vi "MODBUS  SLAVE.vi"() -> (3 "values to write":u16[](array[numeric]) caption="待写入值")   [LabVIEW 2016]
uses:
  <vilib>/NI/Modbus Library/Data Model/Device Data Model.lvclass
  <vilib>/NI/Modbus Library/API/Wrapper/Create TCP Slave.vi
  <vilib>/NI/Modbus Library/API/slave/Modbus Slave.lvclass
  <vilib>/ptbypt/NI_PtbyPt.lvlib
  <vilib>/NI/Modbus Library/API/Wrapper/API Main.lvlib
panel:
  out "运行周期":u16[](array[numeric])
  in  "write operation starting address":u16=100 caption="写操作起始地址"
  out "单仪器启动命令":u16[](array[numeric])
  out "系统启动命令":u16[](array[numeric])
  in  "停止":bool
  out "register values":u16[](array[numeric]) caption="寄存器值"
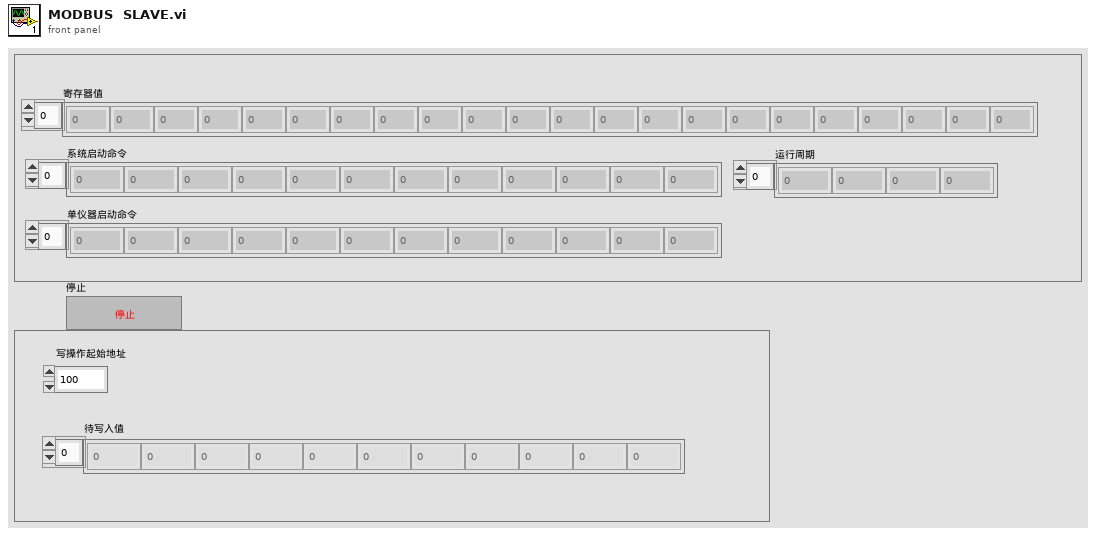
[diagram p1: front panel]
types:
  T1 = cluster{"测量量程":dbl, "测量精度":dbl, "测量间隔":dbl, "消解温度":dbl, "消解时长":dbl, "空白校准时间":timestamp, "曲线截距":dbl, "曲线斜率":dbl, "测量检出限":dbl, "测量信号值":dbl, "线性相关系数":dbl, "二次多项式系数":dbl, "标样校准时间":timestamp, "单位":u16}
  T2 = typedef "LVDateTimeRec.ctl" = cluster{"秒数的小数部分":dbl, "秒":i32, "分":i32, "时":i32, "日":i32, "月":i32, "年":i32, "天数（周）":i32, "天数（年）":i32, "DST":i32}
  T3 = cluster{"时间标识":timestamp, "设备":string, "日志信息":string, "流程参数":string}
  T4 = cluster{"测量模式":enum16{"水样测量", "标样核查", "零点核查", "跨度核查", "空白测试", "加标回收", "平行样", "校零", "校标"}}
  T5 = cluster{"站号":u16, "量程切换":enum32{"H", "L", "AUTO"}, "控制命令":enum16{"启动测量", "标样核查", "零点核查", "跨度核查", "空白测试", "平行样测试", "加标回收", "空白校准", "标样校准", "初始化（清洗）", "停止测试", "仪器重启", "校时", "模式设置", "测量间隔设置"}, "模式设置":enum16{"待机", "连续模式", "周期模式", "定点模式", "受控模式", "手动模式"}, "测量间隔":u16}
  T6 = cluster{"是否启用仪器":bool, "CODMn":cluster{"启动测量模式":cluster{"测量模式":enum16{"水样测量", "标样核查", "加标回收", "平行样", "校零", "校标"}}, "确定按钮":bool}, "启动模块":cluster{"氨氮":bool, "总磷":bool, "总氮":bool, "COD":bool}, "常规启动":bool, "直接启动":bool}
  T7 = cluster{"系统时间":timestamp, "工作状态":enum16{"空闲", "水样测试", "标样核查", "零点核查", "跨度核查", "空白测试", "平行样测试", "加标回收", "空白校准", "标样校准", "初始化（清洗）"}, "测量模式":enum16{"待机", "连续模式", "周期模式", "定点模式", "受控模式", "手动模式"}, "告警代码":u16, "故障代码":u16, "日志代码":u16, "软件版本":u16, "F0":sgl, "F1":sgl, "F2":sgl, "F3":sgl, "T":sgl, "H":sgl, "id":u16, "flowid":u16, "量程":u16, "总磷控温温度1":sgl, "营养盐控温温度2":sgl, "ADC":sgl}
  T8 = enum16{"空闲", "水样测试", "标样核查", "零点核查", "跨度核查", "空白测试", "平行样测试", "质控样", "空白校准", "标样校准", "加标回收"}
  T9 = enum16{"空闲", "水样测试", "标样核查", "零点核查", "跨度核查", "空白测试", "平行样测试", "加标回收", "空白校准", "标样校准", "初始化（清洗）"}
  T10 = cluster{"水样测试量程模式":enum16{"H", "L", "AUTO"}, "空白核查量程模式":enum16{"H", "L", "AUTO"}, "跨度核查量程模式":enum16{"H", "L", "AUTO"}}
  T11 = enum32{"Bad", "Idle", "Run top level", "Running"}
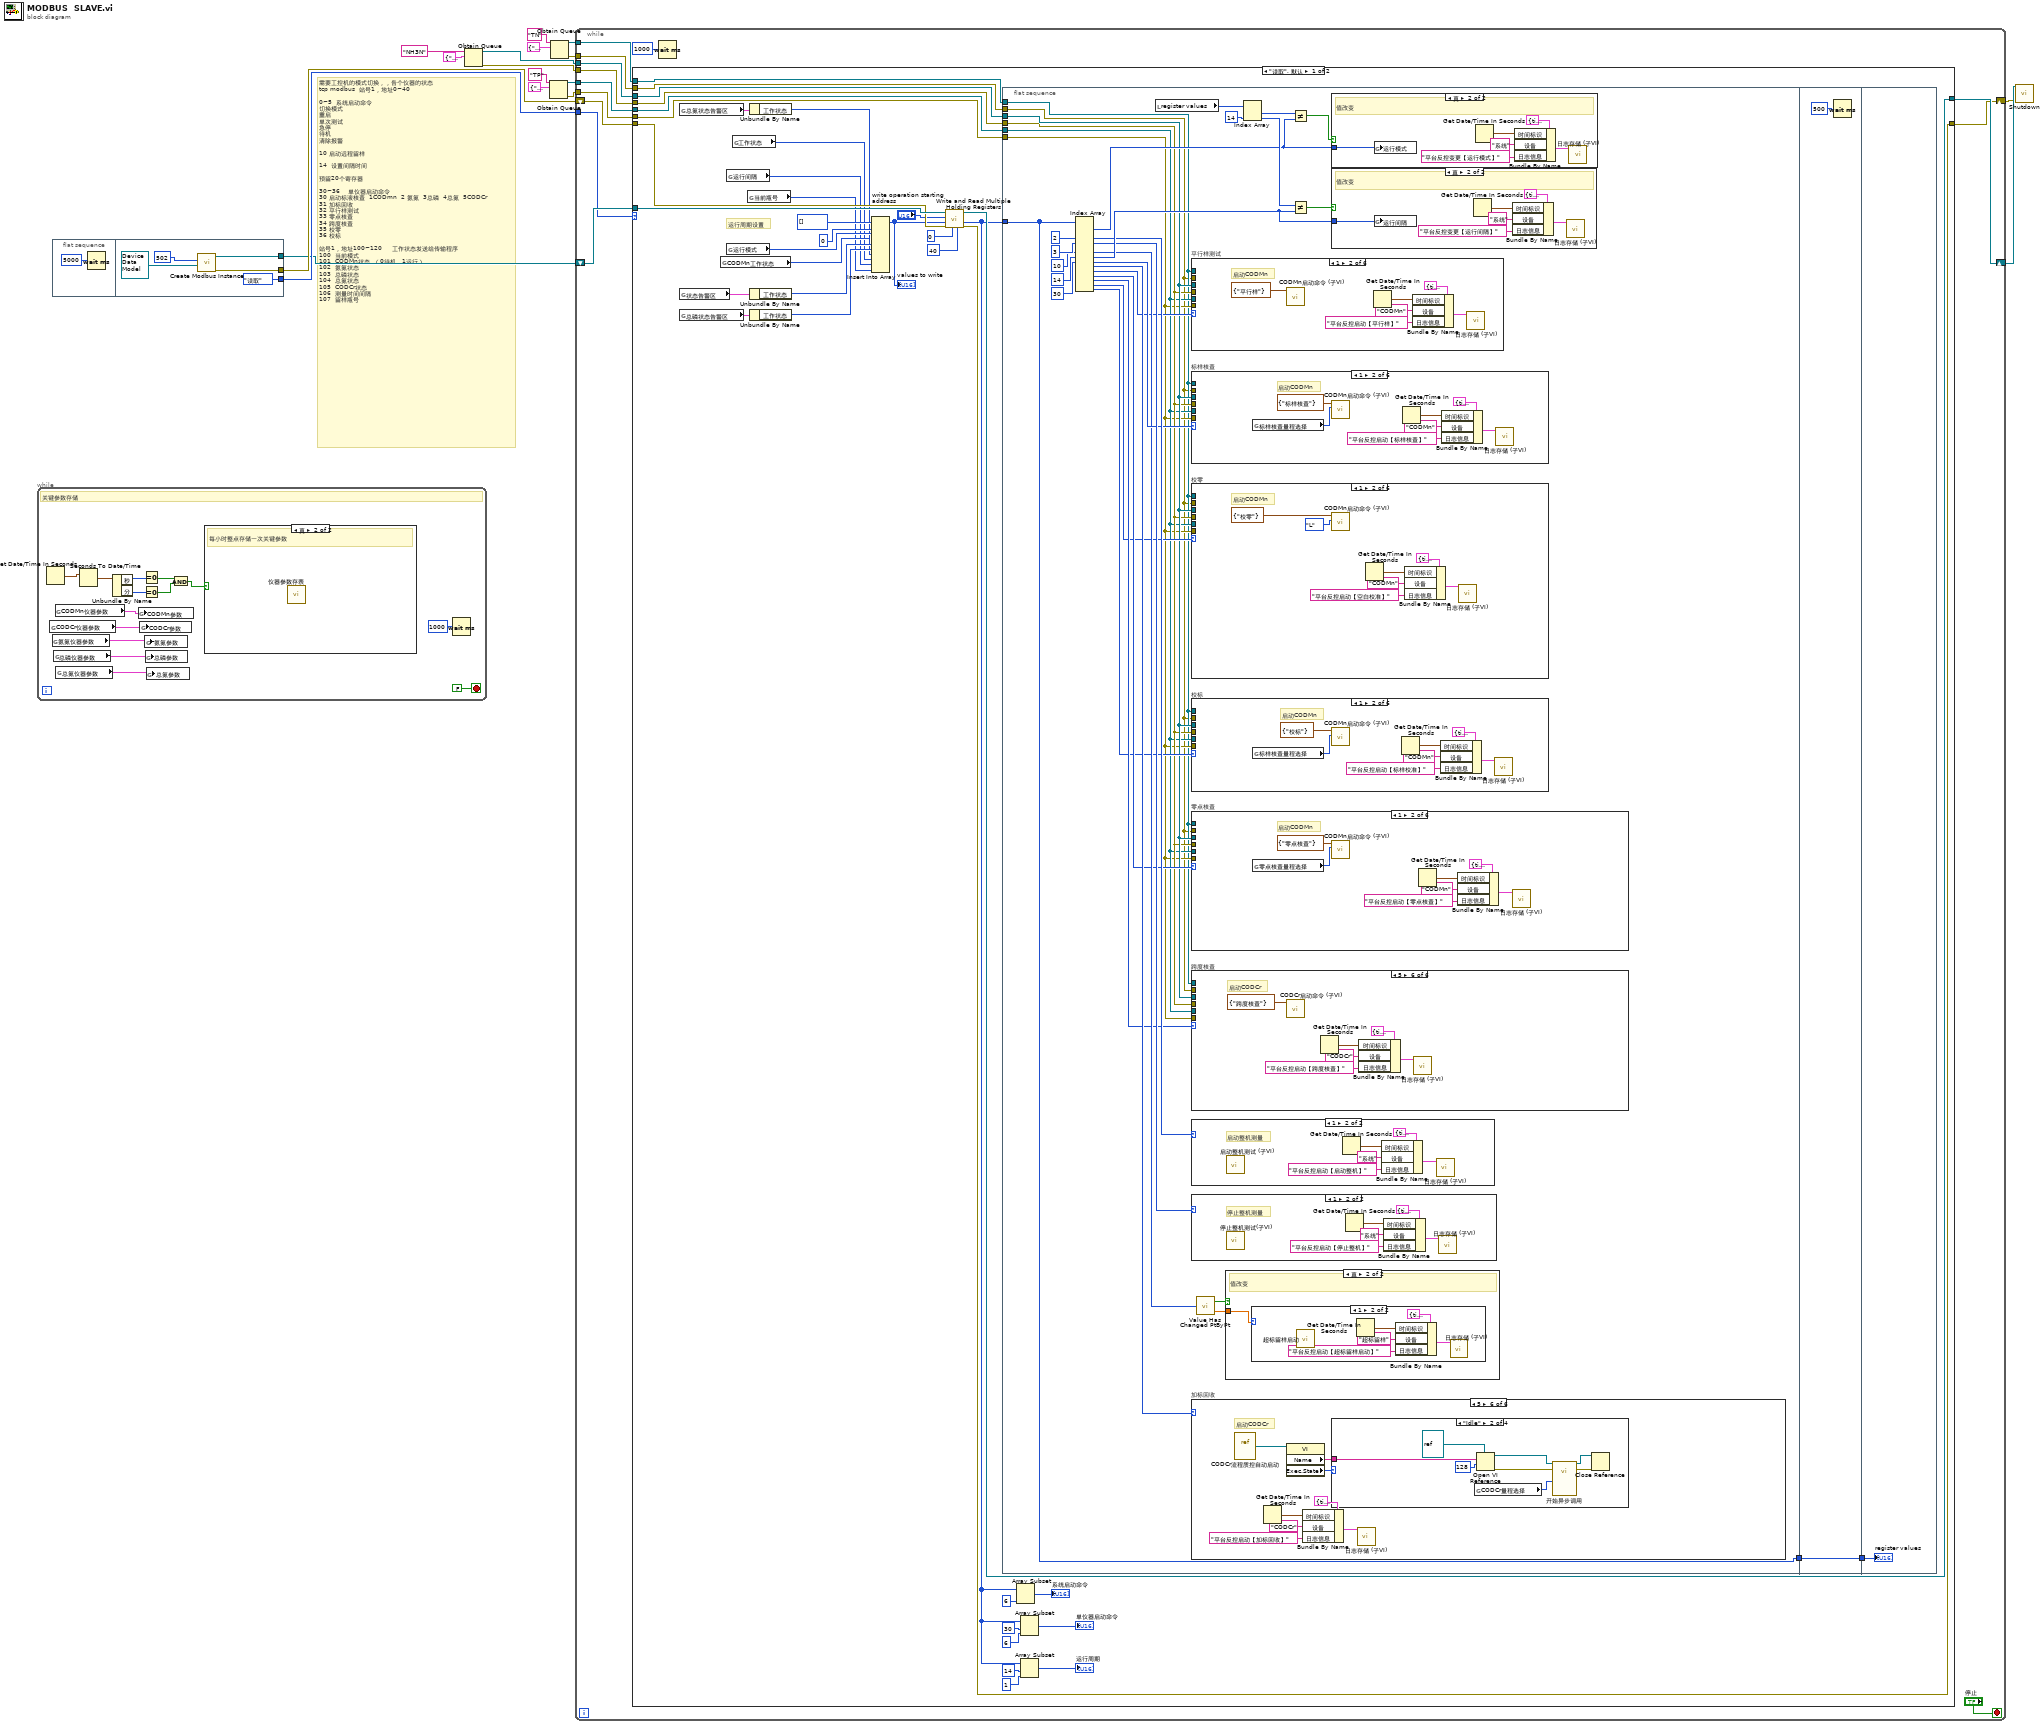
[diagram p0: block diagram]
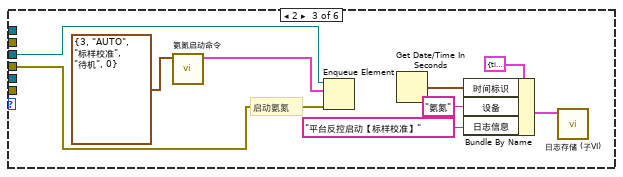
[diagram p4: hidden frame]
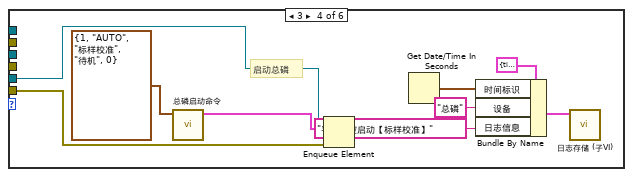
[diagram p5: hidden frame]
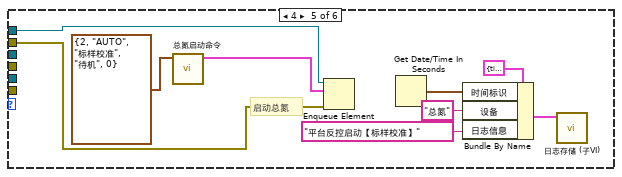
[diagram p6: hidden frame]
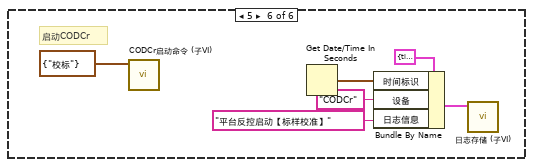
[diagram p7: hidden frame]
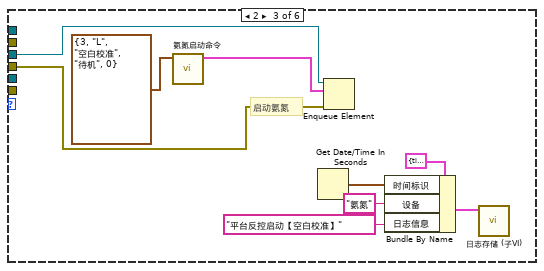
[diagram p9: hidden frame]
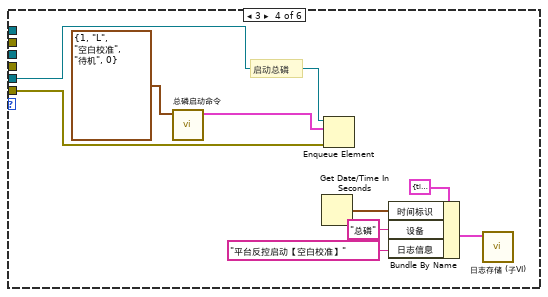
[diagram p10: hidden frame]
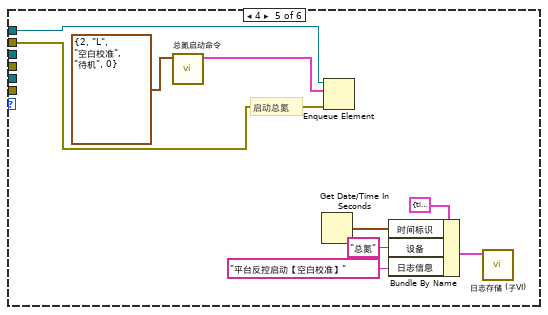
[diagram p11: hidden frame]
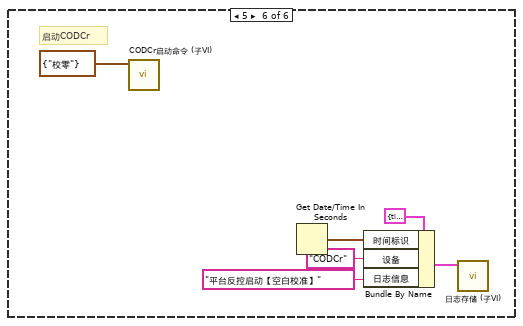
[diagram p12: hidden frame]
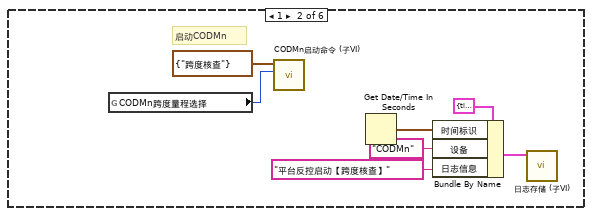
[diagram p14: hidden frame]
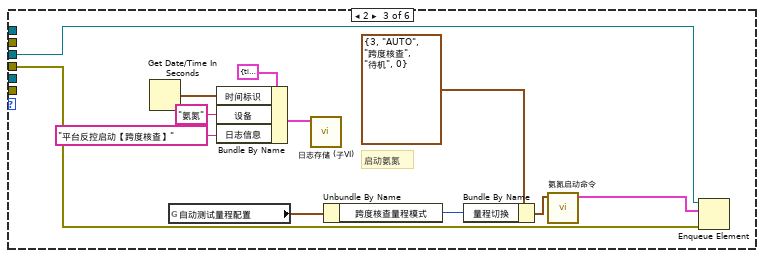
[diagram p15: hidden frame]
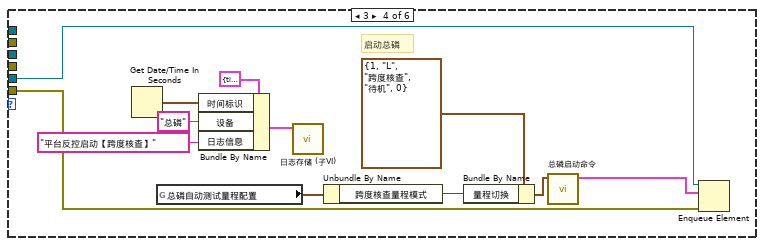
[diagram p16: hidden frame]
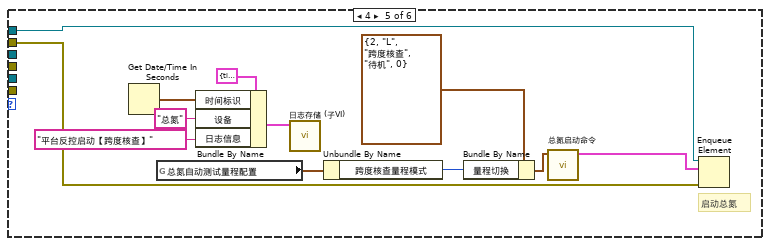
[diagram p17: hidden frame]
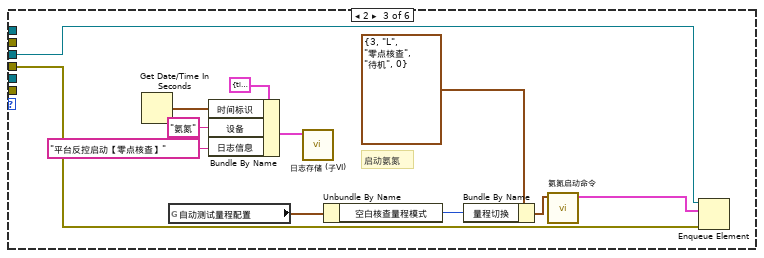
[diagram p19: hidden frame]
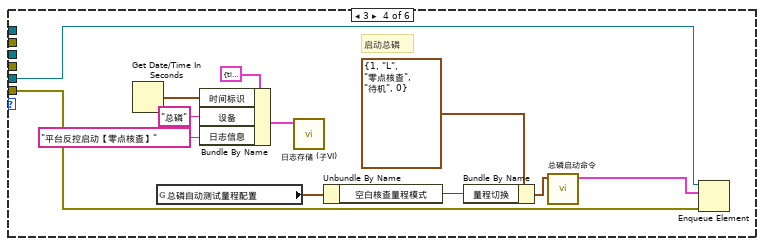
[diagram p20: hidden frame]
diagram:
  # "需要工控机的模式切换，，各个仪器的状态\ntcp modbus  站号1，地址0~40\n\n0~5  系统启动命令\n切换模式\n重启\n单次测试\n急停\n待机\n清除报警\n\n10 启动远程留样\n\n14  设置间隔时间\n\n预留20个寄存器\n\n30~36    单仪器启动命令\n30 启动标液核查  1CODmn  2 氨氮  3总磷  4总氮  5CODCr\n31 加标回收\n32 平行样测试\n33 零点核查\n34 跨度核查\n35 校零\n36 校标\n\n站号1，地址100~120     工作状态发送给传输程序\n100  当前模式\n101  CODMn状态  （0待机，1运行）\n102  氨氮状态\n103  总磷状态\n104  总氮状态\n105  CODCr状态\n106  测量时间间隔\n107  留样瓶号"
  n1 = while {
    stop <- FALSE stop-if-true
    # "关键参数存储"
    n2 = Get Date/Time In Seconds() -> (seconds since 1Jan1904=w29:timestamp)
    n3 = global read "CODcr全局变量.vi" "CODCr仪器参数"() -> (w21:T1)
    n4 = global read "氨氮断电保存全局变量.vi" "氨氮仪器参数"() -> (w20:T1)
    n5 = global read "总磷断电保存全局变量.vi" "总磷仪器参数"() -> (w19:T1)
    n6 = global read "CODMn断电保存全局变量.vi" "CODMn仪器参数"() -> (w22:T1)
    n7 = global read "总氮断电保存全局变量.vi" "总氮仪器参数"() -> (w18:T1)
    n8 = Seconds To Date/Time(time stamp (now)=w29) -> (date time rec=w28:T2)  [unwired: 1 in]
    n9 = Unbundle By Name(w28) -> ("秒"=w27:i32, "分"=w26:i32)
    n10 = global write "在线监测仪器仪表参数.vi" "CODMn参数"(w22) -> ()
    n11 = global write "在线监测仪器仪表参数.vi" "CODCr参数"(w21) -> ()
    n12 = Equal To 0?(x=w27) -> (x = 0?=w25:bool)
    n13 = Equal To 0?(x=w26) -> (x = 0?=w24:bool)
    n14 = global write "在线监测仪器仪表参数.vi" "氨氮参数"(w20) -> ()
    n15 = global write "在线监测仪器仪表参数.vi" "总磷参数"(w19) -> ()
    n16 = global write "在线监测仪器仪表参数.vi" "总氮参数"(w18) -> ()
    n17 = And(x=w25, y=w24) -> (x .and. y?=w23:bool)
    n18 = case shown="真" w23 {
      frame False {
      }
      frame True {
        # "每小时整点存储一次关键参数"
        n19 = call "仪器参数存表.vi"() -> ()  [unwired: 12 in]
      }
    }
    n20 = Wait (ms)(milliseconds to wait=u32 1000 ("等待时间（毫秒）")) -> ()  [unwired: 1 out]
  }
  n21 = flat-sequence {
    tunnel: [enum16{"读取", "写入"}."读取"] -> w17
    tunnel: [w35] -> w16
    tunnel: [w34] -> w15
    frame #0 {
      n22 = Wait (ms)(milliseconds to wait=u32 5000 ("等待时间（毫秒）")) -> ()  [unwired: 1 out]
    }
    frame #1 {
      n23 = call-poly <vilib>:"Create Modbus Instance.vi"("device data model"=refnum<class "Device Data Model.lvclass"> refnum, "port (502)"=u16 502) -> ("error out"=w35:errorcluster, "TCP slave instance"=w34:refnum<class "Modbus Slave.lvclass">)  [unwired: 8 in]
    }
  }
  n24 = Obtain Queue(name (unnamed)="NH3N" ("名称（未命名）"), element data type=cluster{"命令":string, "data":variant} {"命令"="", "data"=variant}) -> (queue out=w6:refnum<queue>, error out=w5:errorcluster)  [unwired: 3 in, 1 out]
  n25 = Obtain Queue(name (unnamed)="TP" ("名称（未命名）"), element data type=cluster{"命令":string, "data":variant} {"命令"="", "data"=variant}) -> (queue out=w4:refnum<queue>, error out=w3:errorcluster)  [unwired: 3 in, 1 out]
  n26 = Obtain Queue(name (unnamed)="TN" ("名称（未命名）"), element data type=cluster{"命令":string, "data":variant} {"命令"="", "data"=variant}) -> (queue out=w2:refnum<queue>, error out=w1:errorcluster)  [unwired: 3 in, 1 out]
  n27 = while {
    shift-right: [w48] -> w14
    shift-left: w15 -> [w50]
    shift-right: [w44] -> w13
    shift-left: w16 -> [w49]
    tunnel: w17 -> [w45]
    tunnel: w6 -> [w43]
    tunnel: w5 -> [w42]
    tunnel: w4 -> [w41]
    tunnel: w3 -> [w40]
    tunnel: w2 -> [w39]
    tunnel: w1 -> [w38]
    stop <- "停止" stop-if-true
    n28 = case shown="\"读取\", 默认" w45 {
      tunnel: w50 -> [w84 w498]
      tunnel: w49 -> [w83 w497]
      tunnel: [w79 w498] -> w48
      tunnel: [w80 w497] -> w44
      tunnel: w43 -> [w56 _]
      tunnel: w42 -> [w55 _]
      tunnel: w41 -> [w54 _]
      tunnel: w40 -> [w53 _]
      tunnel: w39 -> [w52 _]
      tunnel: w38 -> [w51 _]
      frame "读取", Default {
        # "运行周期设置"
        n29 = global read "VAR总磷全局变量.vi" "总氮状态告警区"() -> (w62:T7)
        n30 = global read "VAR氨氮全局变量.vi" "状态告警区"() -> (w66:T7)
        n31 = global read "VAR总磷全局变量.vi" "总磷状态告警区"() -> (w64:T7)
        n32 = global read "COD测量模式全局.vi" "CODMn工作状态"() -> (w60:T8)
        n33 = global read "系统设置全局变量.vi" "运行间隔"() -> (w58:i16)
        n34 = global read "系统设置全局变量.vi" "运行模式"() -> (w76:enum16{"维护模式", "常规模式", "应急模式", "质控模式"})
        n35 = global read "CODcr全局变量.vi" "工作状态"() -> (w59:T9)
        n36 = global read "超标留样全局.vi" "当前瓶号"() -> (w57:u16)
        n37 = Unbundle By Name(w62) -> ("工作状态"=w61:T9)
        n38 = Unbundle By Name(w66) -> ("工作状态"=w65:T9)
        n39 = Unbundle By Name(w64) -> ("工作状态"=w63:T9)
        n40 = Insert Into Array(array=u16[] [] ("values to write"), index=0 ("索引"), new element #1=w76, new element #2=w60, new element #3=w65, new element #4=w63, new element #5=w61, new element #6=w59, new element #7=w58, new element #8=w57) -> (w74:u16[])
        "values to write" <- w74
        n41 = call-dynamic "Write and Read Multiple Holding Registers.vi"("read count"=u16 40 ("number of holding registers"), "read starting address"=u16 0 ("starting address"), "error in"=w83, "write values"=w74, "write starting address"="write operation starting address", "Modbus instance in"=w84) -> ("error out"=w80:errorcluster, "read values"=w69:u16[], "Modbus instance out"=w79:refnum<class "Modbus Slave.lvclass">)  [unwired: 3 in]
        n42 = flat-sequence {
          tunnel: w69 -> [w120]
          tunnel: [w120] -> w68
          tunnel: w56 -> [w94]
          tunnel: w55 -> [w93]
          tunnel: w54 -> [w92]
          tunnel: w53 -> [w91]
          tunnel: w52 -> [w90]
          tunnel: w51 -> [w89]
          tunnel: w68 -> [w494]
          tunnel: [w494] -> w67
          tunnel: w67 -> [w496]
          frame #0 {
            n43 = Index Array(array=w120, index #3=2 ("索引"), index #4=3 ("索引"), index #6=10 ("索引"), index #7=14 ("索引"), index #8=30 ("索引")) -> (element #1=w107:u16, element #3=w108:u16, element #4=w109:u16, element #6=w102:u16, element #7=w110:u16, element #8=w105:u16, element #9=w104:u16, element #10=w99:u16, element #11=w98:u16, element #12=w97:u16, element #13=w96:u16, element #14=w95:u16)  [unwired: 9 in, 2 out]
            n44 = local read "register values"() -> (w119:u16[])
            n45 = case "平行样测试" shown="1" w99 {
              tunnel: w94 -> [_ _ w311 _ _ _]
              tunnel: w93 -> [_ _ w310 _ _ _]
              tunnel: w92 -> [_ _ _ w320 _ _]
              tunnel: w91 -> [_ _ _ w319 _ _]
              tunnel: w90 -> [_ _ _ _ w329 _]
              tunnel: w89 -> [_ _ _ _ w328 _]
              frame 0, Default {
              }
              frame 1 {
                # "启动CODMn"
                n46 = call "CODMn启动命令 (子VI).vi"("启动测量模式"=T4 {"测量模式"=enum."平行样"}) -> ()  [unwired: 11 in]
                n47 = Get Date/Time In Seconds() -> (seconds since 1Jan1904=w301:timestamp)
                n48 = Bundle By Name(cluster=T3 {"时间标识"=timestamp(0 s since 1904-01-01), "设备"="", "日志信息"="", "流程参数"=""} ("data in"), "时间标识"=w301, "设备"="CODMn", "日志信息"="平台反控启动【平行样】") -> (w302:T3)
                n49 = call "日志存储 (子VI).vi"("data in"=w302) -> ()  [unwired: 11 in]
              }
              frame 2 {
                # "启动氨氮"
                n50 = call "氨氮启动命令.vi"("参数"=T5 {"站号"=3, "量程切换"=enum."AUTO", "控制命令"=enum."平行样测试", "模式设置"=enum."待机", "测量间隔"=0}) -> ("启动命令"=w312:cluster{"命令":string, "data":variant})  [unwired: 10 in]
                n51 = Get Date/Time In Seconds() -> (seconds since 1Jan1904=w307:timestamp)
                n52 = Bundle By Name(cluster=T3 {"时间标识"=timestamp(0 s since 1904-01-01), "设备"="", "日志信息"="", "流程参数"=""} ("data in"), "时间标识"=w307, "设备"="氨氮", "日志信息"="平台反控启动【平行样】") -> (w308:T3)
                n53 = Enqueue Element(queue=w311, element=w312, error in (no error)=w310) -> ()  [unwired: 1 in, 3 out]
                n54 = call "日志存储 (子VI).vi"("data in"=w308) -> ()  [unwired: 11 in]
              }
              frame 3 {
                # "启动总磷"
                n55 = call "总磷启动命令.vi"("参数"=T5 {"站号"=1, "量程切换"=enum."AUTO", "控制命令"=enum."平行样测试", "模式设置"=enum."待机", "测量间隔"=0}) -> ("启动命令"=w321:cluster{"命令":string, "data":variant})  [unwired: 10 in]
                n56 = Get Date/Time In Seconds() -> (seconds since 1Jan1904=w316:timestamp)
                n57 = Bundle By Name(cluster=T3 {"时间标识"=timestamp(0 s since 1904-01-01), "设备"="", "日志信息"="", "流程参数"=""} ("data in"), "时间标识"=w316, "设备"="总磷", "日志信息"="平台反控启动【平行样】") -> (w317:T3)
                n58 = Enqueue Element(queue=w320, element=w321, error in (no error)=w319) -> ()  [unwired: 1 in, 3 out]
                n59 = call "日志存储 (子VI).vi"("data in"=w317) -> ()  [unwired: 11 in]
              }
              frame 4 {
                # "启动总氮"
                n60 = call "总氮启动命令.vi"("参数"=T5 {"站号"=2, "量程切换"=enum."AUTO", "控制命令"=enum."平行样测试", "模式设置"=enum."待机", "测量间隔"=0}) -> ("启动命令"=w330:cluster{"命令":string, "data":variant})  [unwired: 10 in]
                n61 = Get Date/Time In Seconds() -> (seconds since 1Jan1904=w325:timestamp)
                n62 = Bundle By Name(cluster=T3 {"时间标识"=timestamp(0 s since 1904-01-01), "设备"="", "日志信息"="", "流程参数"=""} ("data in"), "时间标识"=w325, "设备"="总氮", "日志信息"="平台反控启动【平行样】") -> (w326:T3)
                n63 = Enqueue Element(queue=w329, element=w330, error in (no error)=w328) -> ()  [unwired: 1 in, 3 out]
                n64 = call "日志存储 (子VI).vi"("data in"=w326) -> ()  [unwired: 11 in]
              }
              frame 5 {
                # "启动CODCr"
                n65 = call "CODCr启动命令 (子VI).vi"("启动测量模式"=T4 {"测量模式"=enum."平行样"}) -> ()  [unwired: 11 in]
                n66 = Get Date/Time In Seconds() -> (seconds since 1Jan1904=w334:timestamp)
                n67 = Bundle By Name(cluster=T3 {"时间标识"=timestamp(0 s since 1904-01-01), "设备"="", "日志信息"="", "流程参数"=""} ("data in"), "时间标识"=w334, "设备"="CODCr", "日志信息"="平台反控启动【平行样】") -> (w335:T3)
                n68 = call "日志存储 (子VI).vi"("data in"=w335) -> ()  [unwired: 11 in]
              }
            }
            n69 = case "标样核查" shown="1" w105 {
              tunnel: w94 -> [_ _ w445 _ _ _]
              tunnel: w93 -> [_ _ w444 _ _ _]
              tunnel: w92 -> [_ _ _ w454 _ _]
              tunnel: w91 -> [_ _ _ w453 _ _]
              tunnel: w90 -> [_ _ _ _ w463 _]
              tunnel: w89 -> [_ _ _ _ w462 _]
              frame 0, Default {
              }
              frame 1 {
                # "启动CODMn"
                n70 = global read "CODMn断电保存全局变量.vi" "标样核查量程选择"() -> (w437:enum32{"H", "L", "AUTO"})
                n71 = call "CODMn启动命令 (子VI).vi"("CODMn量程切换"=w437, "启动测量模式"=T4 {"测量模式"=enum."标样核查"}) -> ()  [unwired: 10 in]
                n72 = Get Date/Time In Seconds() -> (seconds since 1Jan1904=w434:timestamp)
                n73 = Bundle By Name(cluster=T3 {"时间标识"=timestamp(0 s since 1904-01-01), "设备"="", "日志信息"="", "流程参数"=""} ("data in"), "时间标识"=w434, "设备"="CODMn", "日志信息"="平台反控启动【标样核查】") -> (w435:T3)
                n74 = call "日志存储 (子VI).vi"("data in"=w435) -> ()  [unwired: 11 in]
              }
              frame 2 {
                # "启动氨氮"
                n75 = call "氨氮启动命令.vi"("参数"=T5 {"站号"=3, "量程切换"=enum."AUTO", "控制命令"=enum."标样核查", "模式设置"=enum."待机", "测量间隔"=0}) -> ("启动命令"=w446:cluster{"命令":string, "data":variant})  [unwired: 10 in]
                n76 = Enqueue Element(queue=w445, element=w446, error in (no error)=w444) -> ()  [unwired: 1 in, 3 out]
                n77 = Get Date/Time In Seconds() -> (seconds since 1Jan1904=w441:timestamp)
                n78 = Bundle By Name(cluster=T3 {"时间标识"=timestamp(0 s since 1904-01-01), "设备"="", "日志信息"="", "流程参数"=""} ("data in"), "时间标识"=w441, "设备"="氨氮", "日志信息"="平台反控启动【标样核查】") -> (w442:T3)
                n79 = call "日志存储 (子VI).vi"("data in"=w442) -> ()  [unwired: 11 in]
              }
              frame 3 {
                # "启动总磷"
                n80 = call "总磷启动命令.vi"("参数"=T5 {"站号"=1, "量程切换"=enum."AUTO", "控制命令"=enum."标样核查", "模式设置"=enum."待机", "测量间隔"=0}) -> ("启动命令"=w455:cluster{"命令":string, "data":variant})  [unwired: 10 in]
                n81 = Enqueue Element(queue=w454, element=w455, error in (no error)=w453) -> ()  [unwired: 1 in, 3 out]
                n82 = Get Date/Time In Seconds() -> (seconds since 1Jan1904=w450:timestamp)
                n83 = Bundle By Name(cluster=T3 {"时间标识"=timestamp(0 s since 1904-01-01), "设备"="", "日志信息"="", "流程参数"=""} ("data in"), "时间标识"=w450, "设备"="总磷", "日志信息"="平台反控启动【标样核查】") -> (w451:T3)
                n84 = call "日志存储 (子VI).vi"("data in"=w451) -> ()  [unwired: 11 in]
              }
              frame 4 {
                # "启动总氮"
                n85 = call "总氮启动命令.vi"("参数"=T5 {"站号"=2, "量程切换"=enum."AUTO", "控制命令"=enum."标样核查", "模式设置"=enum."待机", "测量间隔"=0}) -> ("启动命令"=w464:cluster{"命令":string, "data":variant})  [unwired: 10 in]
                n86 = Enqueue Element(queue=w463, element=w464, error in (no error)=w462) -> ()  [unwired: 1 in, 3 out]
                n87 = Get Date/Time In Seconds() -> (seconds since 1Jan1904=w459:timestamp)
                n88 = Bundle By Name(cluster=T3 {"时间标识"=timestamp(0 s since 1904-01-01), "设备"="", "日志信息"="", "流程参数"=""} ("data in"), "时间标识"=w459, "设备"="总氮", "日志信息"="平台反控启动【标样核查】") -> (w460:T3)
                n89 = call "日志存储 (子VI).vi"("data in"=w460) -> ()  [unwired: 11 in]
              }
              frame 5 {
                # "启动CODCr"
                n90 = call "CODCr启动命令 (子VI).vi"("启动测量模式"=T4 {"测量模式"=enum."标样核查"}) -> ()  [unwired: 11 in]
                n91 = Get Date/Time In Seconds() -> (seconds since 1Jan1904=w468:timestamp)
                n92 = Bundle By Name(cluster=T3 {"时间标识"=timestamp(0 s since 1904-01-01), "设备"="", "日志信息"="", "流程参数"=""} ("data in"), "时间标识"=w468, "设备"="CODCr", "日志信息"="平台反控启动【标样核查】") -> (w469:T3)
                n93 = call "日志存储 (子VI).vi"("data in"=w469) -> ()  [unwired: 11 in]
              }
            }
            n94 = case "校零" shown="1" w96 {
              tunnel: w94 -> [_ _ w174 _ _ _]
              tunnel: w93 -> [_ _ w173 _ _ _]
              tunnel: w92 -> [_ _ _ w183 _ _]
              tunnel: w91 -> [_ _ _ w182 _ _]
              tunnel: w90 -> [_ _ _ _ w192 _]
              tunnel: w89 -> [_ _ _ _ w191 _]
              frame 0, Default {
              }
              frame 1 {
                # "启动CODMn"
                n95 = call "CODMn启动命令 (子VI).vi"("CODMn量程切换"=enum32{"H", "L", "AUTO"}."L", "启动测量模式"=T4 {"测量模式"=enum."校零"}) -> ()  [unwired: 10 in]
                n96 = Get Date/Time In Seconds() -> (seconds since 1Jan1904=w163:timestamp)
                n97 = Bundle By Name(cluster=T3 {"时间标识"=timestamp(0 s since 1904-01-01), "设备"="", "日志信息"="", "流程参数"=""} ("data in"), "时间标识"=w163, "设备"="CODMn", "日志信息"="平台反控启动【空白校准】") -> (w164:T3)
                n98 = call "日志存储 (子VI).vi"("data in"=w164) -> ()  [unwired: 11 in]
              }
              frame 2 {
                # "启动氨氮"
                n99 = call "氨氮启动命令.vi"("参数"=T5 {"站号"=3, "量程切换"=enum."L", "控制命令"=enum."空白校准", "模式设置"=enum."待机", "测量间隔"=0}) -> ("启动命令"=w175:cluster{"命令":string, "data":variant})  [unwired: 10 in]
                n100 = Get Date/Time In Seconds() -> (seconds since 1Jan1904=w170:timestamp)
                n101 = Enqueue Element(queue=w174, element=w175, error in (no error)=w173) -> ()  [unwired: 1 in, 3 out]
                n102 = Bundle By Name(cluster=T3 {"时间标识"=timestamp(0 s since 1904-01-01), "设备"="", "日志信息"="", "流程参数"=""} ("data in"), "时间标识"=w170, "设备"="氨氮", "日志信息"="平台反控启动【空白校准】") -> (w171:T3)
                n103 = call "日志存储 (子VI).vi"("data in"=w171) -> ()  [unwired: 11 in]
              }
              frame 3 {
                # "启动总磷"
                n104 = call "总磷启动命令.vi"("参数"=T5 {"站号"=1, "量程切换"=enum."L", "控制命令"=enum."空白校准", "模式设置"=enum."待机", "测量间隔"=0}) -> ("启动命令"=w184:cluster{"命令":string, "data":variant})  [unwired: 10 in]
                n105 = Get Date/Time In Seconds() -> (seconds since 1Jan1904=w179:timestamp)
                n106 = Enqueue Element(queue=w183, element=w184, error in (no error)=w182) -> ()  [unwired: 1 in, 3 out]
                n107 = Bundle By Name(cluster=T3 {"时间标识"=timestamp(0 s since 1904-01-01), "设备"="", "日志信息"="", "流程参数"=""} ("data in"), "时间标识"=w179, "设备"="总磷", "日志信息"="平台反控启动【空白校准】") -> (w180:T3)
                n108 = call "日志存储 (子VI).vi"("data in"=w180) -> ()  [unwired: 11 in]
              }
              frame 4 {
                # "启动总氮"
                n109 = call "总氮启动命令.vi"("参数"=T5 {"站号"=2, "量程切换"=enum."L", "控制命令"=enum."空白校准", "模式设置"=enum."待机", "测量间隔"=0}) -> ("启动命令"=w193:cluster{"命令":string, "data":variant})  [unwired: 10 in]
                n110 = Get Date/Time In Seconds() -> (seconds since 1Jan1904=w188:timestamp)
                n111 = Enqueue Element(queue=w192, element=w193, error in (no error)=w191) -> ()  [unwired: 1 in, 3 out]
                n112 = Bundle By Name(cluster=T3 {"时间标识"=timestamp(0 s since 1904-01-01), "设备"="", "日志信息"="", "流程参数"=""} ("data in"), "时间标识"=w188, "设备"="总氮", "日志信息"="平台反控启动【空白校准】") -> (w189:T3)
                n113 = call "日志存储 (子VI).vi"("data in"=w189) -> ()  [unwired: 11 in]
              }
              frame 5 {
                # "启动CODCr"
                n114 = call "CODCr启动命令 (子VI).vi"("启动测量模式"=T4 {"测量模式"=enum."校零"}) -> ()  [unwired: 11 in]
                n115 = Get Date/Time In Seconds() -> (seconds since 1Jan1904=w197:timestamp)
                n116 = Bundle By Name(cluster=T3 {"时间标识"=timestamp(0 s since 1904-01-01), "设备"="", "日志信息"="", "流程参数"=""} ("data in"), "时间标识"=w197, "设备"="CODCr", "日志信息"="平台反控启动【空白校准】") -> (w198:T3)
                n117 = call "日志存储 (子VI).vi"("data in"=w198) -> ()  [unwired: 11 in]
              }
            }
            n118 = case "校标" shown="1" w95 {
              tunnel: w94 -> [_ _ w134 _ _ _]
              tunnel: w93 -> [_ _ w133 _ _ _]
              tunnel: w92 -> [_ _ _ w143 _ _]
              tunnel: w91 -> [_ _ _ w142 _ _]
              tunnel: w90 -> [_ _ _ _ w152 _]
              tunnel: w89 -> [_ _ _ _ w151 _]
              frame 0, Default {
              }
              frame 1 {
                # "启动CODMn"
                n119 = global read "CODMn断电保存全局变量.vi" "标样核查量程选择"() -> (w126:enum32{"H", "L", "AUTO"})
                n120 = call "CODMn启动命令 (子VI).vi"("CODMn量程切换"=w126, "启动测量模式"=T4 {"测量模式"=enum."校标"}) -> ()  [unwired: 10 in]
                n121 = Get Date/Time In Seconds() -> (seconds since 1Jan1904=w123:timestamp)
                n122 = Bundle By Name(cluster=T3 {"时间标识"=timestamp(0 s since 1904-01-01), "设备"="", "日志信息"="", "流程参数"=""} ("data in"), "时间标识"=w123, "设备"="CODMn", "日志信息"="平台反控启动【标样校准】") -> (w124:T3)
                n123 = call "日志存储 (子VI).vi"("data in"=w124) -> ()  [unwired: 11 in]
              }
              frame 2 {
                # "启动氨氮"
                n124 = call "氨氮启动命令.vi"("参数"=T5 {"站号"=3, "量程切换"=enum."AUTO", "控制命令"=enum."标样校准", "模式设置"=enum."待机", "测量间隔"=0}) -> ("启动命令"=w135:cluster{"命令":string, "data":variant})  [unwired: 10 in]
                n125 = Enqueue Element(queue=w134, element=w135, error in (no error)=w133) -> ()  [unwired: 1 in, 3 out]
                n126 = Get Date/Time In Seconds() -> (seconds since 1Jan1904=w130:timestamp)
                n127 = Bundle By Name(cluster=T3 {"时间标识"=timestamp(0 s since 1904-01-01), "设备"="", "日志信息"="", "流程参数"=""} ("data in"), "时间标识"=w130, "设备"="氨氮", "日志信息"="平台反控启动【标样校准】") -> (w131:T3)
                n128 = call "日志存储 (子VI).vi"("data in"=w131) -> ()  [unwired: 11 in]
              }
              frame 3 {
                # "启动总磷"
                n129 = call "总磷启动命令.vi"("参数"=T5 {"站号"=1, "量程切换"=enum."AUTO", "控制命令"=enum."标样校准", "模式设置"=enum."待机", "测量间隔"=0}) -> ("启动命令"=w144:cluster{"命令":string, "data":variant})  [unwired: 10 in]
                n130 = Enqueue Element(queue=w143, element=w144, error in (no error)=w142) -> ()  [unwired: 1 in, 3 out]
                n131 = Get Date/Time In Seconds() -> (seconds since 1Jan1904=w139:timestamp)
                n132 = Bundle By Name(cluster=T3 {"时间标识"=timestamp(0 s since 1904-01-01), "设备"="", "日志信息"="", "流程参数"=""} ("data in"), "时间标识"=w139, "设备"="总磷", "日志信息"="平台反控启动【标样校准】") -> (w140:T3)
                n133 = call "日志存储 (子VI).vi"("data in"=w140) -> ()  [unwired: 11 in]
              }
              frame 4 {
                # "启动总氮"
                n134 = call "总氮启动命令.vi"("参数"=T5 {"站号"=2, "量程切换"=enum."AUTO", "控制命令"=enum."标样校准", "模式设置"=enum."待机", "测量间隔"=0}) -> ("启动命令"=w153:cluster{"命令":string, "data":variant})  [unwired: 10 in]
                n135 = Enqueue Element(queue=w152, element=w153, error in (no error)=w151) -> ()  [unwired: 1 in, 3 out]
                n136 = Get Date/Time In Seconds() -> (seconds since 1Jan1904=w148:timestamp)
                n137 = Bundle By Name(cluster=T3 {"时间标识"=timestamp(0 s since 1904-01-01), "设备"="", "日志信息"="", "流程参数"=""} ("data in"), "时间标识"=w148, "设备"="总氮", "日志信息"="平台反控启动【标样校准】") -> (w149:T3)
                n138 = call "日志存储 (子VI).vi"("data in"=w149) -> ()  [unwired: 11 in]
              }
              frame 5 {
                # "启动CODCr"
                n139 = call "CODCr启动命令 (子VI).vi"("启动测量模式"=T4 {"测量模式"=enum."校标"}) -> ()  [unwired: 11 in]
                n140 = Get Date/Time In Seconds() -> (seconds since 1Jan1904=w157:timestamp)
                n141 = Bundle By Name(cluster=T3 {"时间标识"=timestamp(0 s since 1904-01-01), "设备"="", "日志信息"="", "流程参数"=""} ("data in"), "时间标识"=w157, "设备"="CODCr", "日志信息"="平台反控启动【标样校准】") -> (w158:T3)
                n142 = call "日志存储 (子VI).vi"("data in"=w158) -> ()  [unwired: 11 in]
              }
            }
            n143 = case "零点核查" shown="1" w98 {
              tunnel: w94 -> [_ _ w267 _ _ _]
              tunnel: w93 -> [_ _ w266 _ _ _]
              tunnel: w92 -> [_ _ _ w279 _ _]
              tunnel: w91 -> [_ _ _ w278 _ _]
              tunnel: w90 -> [_ _ _ _ w291 _]
              tunnel: w89 -> [_ _ _ _ w290 _]
              frame 0, Default {
              }
              frame 1 {
                # "启动CODMn"
                n144 = global read "CODMn断电保存全局变量.vi" "零点核查量程选择"() -> (w255:enum32{"H", "L", "AUTO"})
                n145 = call "CODMn启动命令 (子VI).vi"("CODMn量程切换"=w255, "启动测量模式"=T4 {"测量模式"=enum."零点核查"}) -> ()  [unwired: 10 in]
                n146 = Get Date/Time In Seconds() -> (seconds since 1Jan1904=w252:timestamp)
                n147 = Bundle By Name(cluster=T3 {"时间标识"=timestamp(0 s since 1904-01-01), "设备"="", "日志信息"="", "流程参数"=""} ("data in"), "时间标识"=w252, "设备"="CODMn", "日志信息"="平台反控启动【零点核查】") -> (w253:T3)
                n148 = call "日志存储 (子VI).vi"("data in"=w253) -> ()  [unwired: 11 in]
              }
              frame 2 {
                # "启动氨氮"
                n149 = Get Date/Time In Seconds() -> (seconds since 1Jan1904=w259:timestamp)
                n150 = global read "氨氮断电保存全局变量.vi" "自动测试量程配置"() -> (w265:T10)
                n151 = Bundle By Name(cluster=T3 {"时间标识"=timestamp(0 s since 1904-01-01), "设备"="", "日志信息"="", "流程参数"=""} ("data in"), "时间标识"=w259, "设备"="氨氮", "日志信息"="平台反控启动【零点核查】") -> (w260:T3)
                n152 = call "日志存储 (子VI).vi"("data in"=w260) -> ()  [unwired: 11 in]
                n153 = Unbundle By Name(w265) -> ("空白核查量程模式"=w263:enum16{"H", "L", "AUTO"})
                n154 = Bundle By Name(cluster=T5 {"站号"=3, "量程切换"=enum."L", "控制命令"=enum."零点核查", "模式设置"=enum."待机", "测量间隔"=0} ("参数"), "量程切换"=w263) -> (w262:T5)
                n155 = call "氨氮启动命令.vi"("参数"=w262) -> ("启动命令"=w268:cluster{"命令":string, "data":variant})  [unwired: 10 in]
                n156 = Enqueue Element(queue=w267, element=w268, error in (no error)=w266) -> ()  [unwired: 1 in, 3 out]
              }
              frame 3 {
                # "启动总磷"
                n157 = Get Date/Time In Seconds() -> (seconds since 1Jan1904=w271:timestamp)
                n158 = global read "总磷断电保存全局变量.vi" "总磷自动测试量程配置"() -> (w276:T10)
                n159 = Bundle By Name(cluster=T3 {"时间标识"=timestamp(0 s since 1904-01-01), "设备"="", "日志信息"="", "流程参数"=""} ("data in"), "时间标识"=w271, "设备"="总磷", "日志信息"="平台反控启动【零点核查】") -> (w272:T3)
                n160 = call "日志存储 (子VI).vi"("data in"=w272) -> ()  [unwired: 11 in]
                n161 = Unbundle By Name(w276) -> ("空白核查量程模式"=w275:enum16{"H", "L", "AUTO"})
                n162 = Bundle By Name(cluster=T5 {"站号"=1, "量程切换"=enum."L", "控制命令"=enum."零点核查", "模式设置"=enum."待机", "测量间隔"=0} ("参数"), "量程切换"=w275) -> (w274:T5)
                n163 = call "总磷启动命令.vi"("参数"=w274) -> ("启动命令"=w280:cluster{"命令":string, "data":variant})  [unwired: 10 in]
                n164 = Enqueue Element(queue=w279, element=w280, error in (no error)=w278) -> ()  [unwired: 1 in, 3 out]
              }
              frame 4 {
                # "启动总氮"
                n165 = global read "总氮断电保存全局变量.vi" "总氮自动测试量程配置"() -> (w287:T10)
                n166 = Get Date/Time In Seconds() -> (seconds since 1Jan1904=w283:timestamp)
                n167 = Bundle By Name(cluster=T3 {"时间标识"=timestamp(0 s since 1904-01-01), "设备"="", "日志信息"="", "流程参数"=""} ("data in"), "时间标识"=w283, "设备"="总氮", "日志信息"="平台反控启动【零点核查】") -> (w284:T3)
                n168 = Unbundle By Name(w287) -> ("空白核查量程模式"=w286:enum16{"H", "L", "AUTO"})
                n169 = call "日志存储 (子VI).vi"("data in"=w284) -> ()  [unwired: 11 in]
                n170 = Bundle By Name(cluster=T5 {"站号"=2, "量程切换"=enum."L", "控制命令"=enum."零点核查", "模式设置"=enum."待机", "测量间隔"=0} ("参数"), "量程切换"=w286) -> (w288:T5)
                n171 = call "总氮启动命令.vi"("参数"=w288) -> ("启动命令"=w292:cluster{"命令":string, "data":variant})  [unwired: 10 in]
                n172 = Enqueue Element(queue=w291, element=w292, error in (no error)=w290) -> ()  [unwired: 1 in, 3 out]
              }
              frame 5 {
                # "启动CODCr"
                n173 = call "CODCr启动命令 (子VI).vi"("启动测量模式"=T4 {"测量模式"=enum."零点核查"}) -> ()  [unwired: 11 in]
                n174 = Get Date/Time In Seconds() -> (seconds since 1Jan1904=w295:timestamp)
                n175 = Bundle By Name(cluster=T3 {"时间标识"=timestamp(0 s since 1904-01-01), "设备"="", "日志信息"="", "流程参数"=""} ("data in"), "时间标识"=w295, "设备"="CODCr", "日志信息"="平台反控启动【零点核查】") -> (w296:T3)
                n176 = call "日志存储 (子VI).vi"("data in"=w296) -> ()  [unwired: 11 in]
              }
            }
            n177 = case "跨度核查" shown="5" w97 {
              tunnel: w94 -> [_ _ w218 _ _ _]
              tunnel: w93 -> [_ _ w217 _ _ _]
              tunnel: w92 -> [_ _ _ w230 _ _]
              tunnel: w91 -> [_ _ _ w229 _ _]
              tunnel: w90 -> [_ _ _ _ w242 _]
              tunnel: w89 -> [_ _ _ _ w241 _]
              frame 0, Default {
              }
              frame 1 {
                # "启动CODMn"
                n178 = global read "CODMn断电保存全局变量.vi" "CODMn跨度量程选择"() -> (w206:enum32{"H", "L", "AUTO"})
                n179 = call "CODMn启动命令 (子VI).vi"("CODMn量程切换"=w206, "启动测量模式"=T4 {"测量模式"=enum."跨度核查"}) -> ()  [unwired: 10 in]
                n180 = Get Date/Time In Seconds() -> (seconds since 1Jan1904=w203:timestamp)
                n181 = Bundle By Name(cluster=T3 {"时间标识"=timestamp(0 s since 1904-01-01), "设备"="", "日志信息"="", "流程参数"=""} ("data in"), "时间标识"=w203, "设备"="CODMn", "日志信息"="平台反控启动【跨度核查】") -> (w204:T3)
                n182 = call "日志存储 (子VI).vi"("data in"=w204) -> ()  [unwired: 11 in]
              }
              frame 2 {
                # "启动氨氮"
                n183 = Get Date/Time In Seconds() -> (seconds since 1Jan1904=w210:timestamp)
                n184 = global read "氨氮断电保存全局变量.vi" "自动测试量程配置"() -> (w215:T10)
                n185 = Bundle By Name(cluster=T3 {"时间标识"=timestamp(0 s since 1904-01-01), "设备"="", "日志信息"="", "流程参数"=""} ("data in"), "时间标识"=w210, "设备"="氨氮", "日志信息"="平台反控启动【跨度核查】") -> (w211:T3)
                n186 = call "日志存储 (子VI).vi"("data in"=w211) -> ()  [unwired: 11 in]
                n187 = Unbundle By Name(w215) -> ("跨度核查量程模式"=w214:enum16{"H", "L", "AUTO"})
                n188 = Bundle By Name(cluster=T5 {"站号"=3, "量程切换"=enum."AUTO", "控制命令"=enum."跨度核查", "模式设置"=enum."待机", "测量间隔"=0} ("参数"), "量程切换"=w214) -> (w213:T5)
                n189 = call "氨氮启动命令.vi"("参数"=w213) -> ("启动命令"=w219:cluster{"命令":string, "data":variant})  [unwired: 10 in]
                n190 = Enqueue Element(queue=w218, element=w219, error in (no error)=w217) -> ()  [unwired: 1 in, 3 out]
              }
              frame 3 {
                # "启动总磷"
                n191 = Get Date/Time In Seconds() -> (seconds since 1Jan1904=w222:timestamp)
                n192 = global read "总磷断电保存全局变量.vi" "总磷自动测试量程配置"() -> (w226:T10)
                n193 = Bundle By Name(cluster=T3 {"时间标识"=timestamp(0 s since 1904-01-01), "设备"="", "日志信息"="", "流程参数"=""} ("data in"), "时间标识"=w222, "设备"="总磷", "日志信息"="平台反控启动【跨度核查】") -> (w223:T3)
                n194 = call "日志存储 (子VI).vi"("data in"=w223) -> ()  [unwired: 11 in]
                n195 = Unbundle By Name(w226) -> ("跨度核查量程模式"=w225:enum16{"H", "L", "AUTO"})
                n196 = Bundle By Name(cluster=T5 {"站号"=1, "量程切换"=enum."L", "控制命令"=enum."跨度核查", "模式设置"=enum."待机", "测量间隔"=0} ("参数"), "量程切换"=w225) -> (w227:T5)
                n197 = call "总磷启动命令.vi"("参数"=w227) -> ("启动命令"=w231:cluster{"命令":string, "data":variant})  [unwired: 10 in]
                n198 = Enqueue Element(queue=w230, element=w231, error in (no error)=w229) -> ()  [unwired: 1 in, 3 out]
              }
              frame 4 {
                # "启动总氮"
                n199 = Get Date/Time In Seconds() -> (seconds since 1Jan1904=w234:timestamp)
                n200 = global read "总氮断电保存全局变量.vi" "总氮自动测试量程配置"() -> (w239:T10)
                n201 = Bundle By Name(cluster=T3 {"时间标识"=timestamp(0 s since 1904-01-01), "设备"="", "日志信息"="", "流程参数"=""} ("data in"), "时间标识"=w234, "设备"="总氮", "日志信息"="平台反控启动【跨度核查】") -> (w235:T3)
                n202 = call "日志存储 (子VI).vi"("data in"=w235) -> ()  [unwired: 11 in]
                n203 = Unbundle By Name(w239) -> ("跨度核查量程模式"=w237:enum16{"H", "L", "AUTO"})
                n204 = Bundle By Name(cluster=T5 {"站号"=2, "量程切换"=enum."L", "控制命令"=enum."跨度核查", "模式设置"=enum."待机", "测量间隔"=0} ("参数"), "量程切换"=w237) -> (w238:T5)
                n205 = call "总氮启动命令.vi"("参数"=w238) -> ("启动命令"=w243:cluster{"命令":string, "data":variant})  [unwired: 10 in]
                n206 = Enqueue Element(queue=w242, element=w243, error in (no error)=w241) -> ()  [unwired: 1 in, 3 out]
              }
              frame 5 {
                # "启动CODCr"
                n207 = call "CODCr启动命令 (子VI).vi"("启动测量模式"=T4 {"测量模式"=enum."跨度核查"}) -> ()  [unwired: 11 in]
                n208 = Get Date/Time In Seconds() -> (seconds since 1Jan1904=w246:timestamp)
                n209 = Bundle By Name(cluster=T3 {"时间标识"=timestamp(0 s since 1904-01-01), "设备"="", "日志信息"="", "流程参数"=""} ("data in"), "时间标识"=w246, "设备"="CODCr", "日志信息"="平台反控启动【跨度核查】") -> (w247:T3)
                n210 = call "日志存储 (子VI).vi"("data in"=w247) -> ()  [unwired: 11 in]
              }
            }
            n211 = case shown="1" w108 {
              frame 0, Default {
              }
              frame 1 {
                # "启动整机测量"
                n212 = call "启动整机测试 (子VI).vi"() -> ()  [unwired: 12 in]
                n213 = Get Date/Time In Seconds() -> (seconds since 1Jan1904=w491:timestamp)
                n214 = Bundle By Name(cluster=T3 {"时间标识"=timestamp(0 s since 1904-01-01), "设备"="", "日志信息"="", "流程参数"=""} ("data in"), "时间标识"=w491, "设备"="系统", "日志信息"="平台反控启动【启动整机】") -> (w492:T3)
                n215 = call "日志存储 (子VI).vi"("data in"=w492) -> ()  [unwired: 11 in]
              }
            }
            n216 = case shown="1" w109 {
              frame 0, Default {
              }
              frame 1 {
                # "停止整机测量"
                n217 = call "停止整机测试(子VI).vi"() -> ()  [unwired: 12 in]
                n218 = Get Date/Time In Seconds() -> (seconds since 1Jan1904=w486:timestamp)
                n219 = Bundle By Name(cluster=T3 {"时间标识"=timestamp(0 s since 1904-01-01), "设备"="", "日志信息"="", "流程参数"=""} ("data in"), "时间标识"=w486, "设备"="系统", "日志信息"="平台反控启动【停止整机】") -> (w487:T3)
                n220 = call "日志存储 (子VI).vi"("data in"=w487) -> ()  [unwired: 11 in]
              }
            }
            n221 = case "加标回收" shown="5" w104 {
              frame 0, Default {
              }
              frame 1 {
                # "加标回收"
                # "启动CODMn"
                n222 = Get Date/Time In Seconds() -> (seconds since 1Jan1904=w346:timestamp)
                n223 = Bundle By Name(cluster=T3 {"时间标识"=timestamp(0 s since 1904-01-01), "设备"="", "日志信息"="", "流程参数"=""} ("data in"), "时间标识"=w346, "设备"="CODMn", "日志信息"="平台反控启动【加标回收】") -> (w347:T3)
                n224 = vi-ref "质控单元.lvlib:CODMn流程质控自动启动.vi"() -> (w349:refnum<vi>)
                n225 = call "日志存储 (子VI).vi"("data in"=w347) -> ()  [unwired: 11 in]
                n226 = property class="VI"(reference=w349) -> ("Name"=w351:string, "Exec.State"=w350:T11)  [unwired: 1 in, 2 out]
                n227 = case shown="\"Idle\"" w350 {
                  tunnel: w351 -> [_ w355 _ _]
                  frame "Bad", Default {
                  }
                  frame "Idle" {
                    n228 = global read "断电保存全局.vi" "CODMn量程选择"() -> (w352:enum32{"H", "L", "AUTO"})
                    n229 = Open VI Reference(type specifier VI Refnum (for type only)=refnum<vi> refnum ("类型说明符VI引用句柄（仅用于类型）"), vi path=w355, options=128 ("选项")) -> (vi reference=w359:refnum<vi>, error out=w354:errorcluster)  [unwired: 3 in]
                    n230 = call-by-ref "开始异步调用"(reference=w359, error in=w354, "氨氮量程切换"=w352) -> (reference out=w358:refnum<vi>, error out=w353:errorcluster)  [unwired: 11 in]
                    n231 = Close Reference(reference=w358, error in (no error)=w353) -> ()  [unwired: 1 out]
                  }
                  frame "Run top level" {
                  }
                  frame "Running" {
                  }
                }
              }
              frame 2 {
                # "启动氨氮"
                n232 = Get Date/Time In Seconds() -> (seconds since 1Jan1904=w362:timestamp)
                n233 = Bundle By Name(cluster=T3 {"时间标识"=timestamp(0 s since 1904-01-01), "设备"="", "日志信息"="", "流程参数"=""} ("data in"), "时间标识"=w362, "设备"="氨氮", "日志信息"="平台反控启动【加标回收】") -> (w363:T3)
                n234 = vi-ref "质控单元.lvlib:氨氮流程质控自动启动.vi"() -> (w367:refnum<vi>)
                n235 = call "日志存储 (子VI).vi"("data in"=w363) -> ()  [unwired: 11 in]
                n236 = property class="VI"(reference=w367) -> ("Name"=w365:string, "Exec.State"=w366:T11)  [unwired: 1 in, 2 out]
                n237 = case shown="\"Idle\"" w366 {
                  tunnel: w365 -> [_ w371 _ _]
                  frame "Bad", Default {
                  }
                  frame "Idle" {
                    n238 = global read "断电保存全局.vi" "氨氮量程选择"() -> (w368:enum32{"H", "L", "AUTO"})
                    n239 = Open VI Reference(type specifier VI Refnum (for type only)=refnum<vi> refnum ("类型说明符VI引用句柄（仅用于类型）"), vi path=w371, options=128 ("选项")) -> (vi reference=w375:refnum<vi>, error out=w370:errorcluster)  [unwired: 3 in]
                    n240 = call-by-ref "开始异步调用"(reference=w375, error in=w370, "氨氮量程切换"=w368) -> (reference out=w374:refnum<vi>, error out=w369:errorcluster)  [unwired: 11 in]
                    n241 = Close Reference(reference=w374, error in (no error)=w369) -> ()  [unwired: 1 out]
                  }
                  frame "Run top level" {
                  }
                  frame "Running" {
                  }
                }
              }
              frame 3 {
                # "启动总磷"
                n242 = Get Date/Time In Seconds() -> (seconds since 1Jan1904=w378:timestamp)
                n243 = Bundle By Name(cluster=T3 {"时间标识"=timestamp(0 s since 1904-01-01), "设备"="", "日志信息"="", "流程参数"=""} ("data in"), "时间标识"=w378, "设备"="总磷", "日志信息"="平台反控启动【加标回收】") -> (w379:T3)
                n244 = vi-ref "质控单元.lvlib:总磷流程质控自动启动.vi"() -> (w383:refnum<vi>)
                n245 = call "日志存储 (子VI).vi"("data in"=w379) -> ()  [unwired: 11 in]
                n246 = property class="VI"(reference=w383) -> ("Name"=w382:string, "Exec.State"=w381:T11)  [unwired: 1 in, 2 out]
                n247 = case shown="\"Idle\"" w381 {
                  tunnel: w382 -> [_ w391 _ _]
                  frame "Bad", Default {
                  }
                  frame "Idle" {
                    n248 = Bundle By Name(cluster=T6 {"是否启用仪器"=FALSE, "CODMn"={"启动测量模式"={"测量模式"=enum."水样测量"}, "确定按钮"=FALSE}, "启动模块"={"氨氮"=FALSE, "总磷"=FALSE, "总氮"=FALSE, "COD"=FALSE}, "常规启动"=FALSE, "直接启动"=FALSE} ("参数"), "启动模块.总磷"=TRUE, "启动模块.总氮"=FALSE) -> (w387:T6)
                    n249 = global read "断电保存全局.vi" "总磷量程选择"() -> (w384:enum32{"H", "L", "AUTO"})
                    n250 = Open VI Reference(type specifier VI Refnum (for type only)=refnum<vi> refnum ("类型说明符VI引用句柄（仅用于类型）"), vi path=w391, options=128 ("选项")) -> (vi reference=w395:refnum<vi>, error out=w389:errorcluster)  [unwired: 3 in]
                    n251 = call-by-ref "开始异步调用"(reference=w395, error in=w389, "总磷量程切换"=w384, "参数"=w387) -> (reference out=w394:refnum<vi>, error out=w390:errorcluster)  [unwired: 10 in]
                    n252 = Close Reference(reference=w394, error in (no error)=w390) -> ()  [unwired: 1 out]
                  }
                  frame "Run top level" {
                  }
                  frame "Running" {
                  }
                }
              }
              frame 4 {
                # "启动总氮"
                n253 = Get Date/Time In Seconds() -> (seconds since 1Jan1904=w398:timestamp)
                n254 = Bundle By Name(cluster=T3 {"时间标识"=timestamp(0 s since 1904-01-01), "设备"="", "日志信息"="", "流程参数"=""} ("data in"), "时间标识"=w398, "设备"="总氮", "日志信息"="平台反控启动【加标回收】") -> (w399:T3)
                n255 = vi-ref "质控单元.lvlib:总氮流程质控自动启动.vi"() -> (w403:refnum<vi>)
                n256 = call "日志存储 (子VI).vi"("data in"=w399) -> ()  [unwired: 11 in]
                n257 = property class="VI"(reference=w403) -> ("Name"=w402:string, "Exec.State"=w401:T11)  [unwired: 1 in, 2 out]
                n258 = case shown="\"Idle\"" w401 {
                  tunnel: w402 -> [_ w411 _ _]
                  frame "Bad", Default {
                  }
                  frame "Idle" {
                    n259 = Bundle By Name(cluster=T6 {"是否启用仪器"=FALSE, "CODMn"={"启动测量模式"={"测量模式"=enum."水样测量"}, "确定按钮"=FALSE}, "启动模块"={"氨氮"=FALSE, "总磷"=FALSE, "总氮"=FALSE, "COD"=FALSE}, "常规启动"=FALSE, "直接启动"=FALSE} ("参数"), "启动模块.总磷"=FALSE, "启动模块.总氮"=TRUE) -> (w407:T6)
                    n260 = global read "断电保存全局.vi" "总氮量程选择"() -> (w404:enum32{"H", "L", "AUTO"})
                    n261 = Open VI Reference(type specifier VI Refnum (for type only)=refnum<vi> refnum ("类型说明符VI引用句柄（仅用于类型）"), vi path=w411, options=128 ("选项")) -> (vi reference=w415:refnum<vi>, error out=w409:errorcluster)  [unwired: 3 in]
                    n262 = call-by-ref "开始异步调用"(reference=w415, error in=w409, "总磷量程切换"=w404, "参数"=w407) -> (reference out=w414:refnum<vi>, error out=w410:errorcluster)  [unwired: 10 in]
                    n263 = Close Reference(reference=w414, error in (no error)=w410) -> ()  [unwired: 1 out]
                  }
                  frame "Run top level" {
                  }
                  frame "Running" {
                  }
                }
              }
              frame 5 {
                # "启动CODCr"
                n264 = vi-ref "CODCr流程质控自动启动.vi"() -> (w423:refnum<vi>)
                n265 = Get Date/Time In Seconds() -> (seconds since 1Jan1904=w418:timestamp)
                n266 = property class="VI"(reference=w423) -> ("Name"=w421:string, "Exec.State"=w422:T11)  [unwired: 1 in, 2 out]
                n267 = Bundle By Name(cluster=T3 {"时间标识"=timestamp(0 s since 1904-01-01), "设备"="", "日志信息"="", "流程参数"=""} ("data in"), "时间标识"=w418, "设备"="CODCr", "日志信息"="平台反控启动【加标回收】") -> (w419:T3)
                n268 = case shown="\"Idle\"" w422 {
                  tunnel: w421 -> [_ w427 _ _]
                  frame "Bad", Default {
                  }
                  frame "Idle" {
                    n269 = global read "断电保存全局.vi" "CODCr量程选择"() -> (w424:enum32{"H", "L", "AUTO"})
                    n270 = Open VI Reference(type specifier VI Refnum (for type only)=refnum<vi> refnum ("类型说明符VI引用句柄（仅用于类型）"), vi path=w427, options=128 ("选项")) -> (vi reference=w431:refnum<vi>, error out=w426:errorcluster)  [unwired: 3 in]
                    n271 = call-by-ref "开始异步调用"(reference=w431, error in=w426, "CODMn量程切换"=w424) -> (reference out=w430:refnum<vi>, error out=w425:errorcluster)  [unwired: 10 in]
                    n272 = Close Reference(reference=w430, error in (no error)=w425) -> ()  [unwired: 1 out]
                  }
                  frame "Run top level" {
                  }
                  frame "Running" {
                  }
                }
                n273 = call "日志存储 (子VI).vi"("data in"=w419) -> ()  [unwired: 11 in]
              }
            }
            n274 = call <vilib>:"Value Has Changed PtByPt.vi"("input data point"=w102) -> ("has changed"=w101:bool, "output data point"=w100:dbl)  [unwired: 1 in]
            n275 = case shown="真" w101 {
              tunnel: w100 -> [_ w338]
              frame False {
              }
              frame True {
                # "值改变"
                n276 = case shown="1" w338 {
                  frame 0, Default {
                  }
                  frame 1 {
                    n277 = call "超标留样启动.vi"() -> ()  [unwired: 11 in, 1 out]
                    n278 = Get Date/Time In Seconds() -> (seconds since 1Jan1904=w341:timestamp)
                    n279 = Bundle By Name(cluster=T3 {"时间标识"=timestamp(0 s since 1904-01-01), "设备"="", "日志信息"="", "流程参数"=""} ("data in"), "时间标识"=w341, "设备"="超标留样", "日志信息"="平台反控启动【超标留样启动】") -> (w342:T3)
                    n280 = call "日志存储 (子VI).vi"("data in"=w342) -> ()  [unwired: 11 in]
                  }
                }
              }
            }
            n281 = Index Array(array=w119, index #2=14 ("索引")) -> (element #1=w118:u16, element #2=w115:u16)  [unwired: 1 in]
            n282 = Not Equal?(x=w118, y=w107) -> (x != y?=w117:bool)
            n283 = Not Equal?(x=w115, y=w110) -> (x != y?=w114:bool)
            n284 = case shown="真" w117 {
              tunnel: w107 -> [_ w483]
              frame False {
              }
              frame True {
                # "值改变"
                n285 = global write "系统设置全局变量.vi" "运行模式"(w483) -> ()
                n286 = Get Date/Time In Seconds() -> (seconds since 1Jan1904=w480:timestamp)
                n287 = Bundle By Name(cluster=T3 {"时间标识"=timestamp(0 s since 1904-01-01), "设备"="", "日志信息"="", "流程参数"=""} ("data in"), "时间标识"=w480, "设备"="系统", "日志信息"="平台反控变更【运行模式】") -> (w481:T3)
                n288 = call "日志存储 (子VI).vi"("data in"=w481) -> ()  [unwired: 11 in]
              }
            }
            n289 = case shown="真" w114 {
              tunnel: w110 -> [_ w477]
              frame False {
              }
              frame True {
                # "值改变"
                n290 = global write "系统设置全局变量.vi" "运行间隔"(w477) -> ()
                n291 = Get Date/Time In Seconds() -> (seconds since 1Jan1904=w474:timestamp)
                n292 = Bundle By Name(cluster=T3 {"时间标识"=timestamp(0 s since 1904-01-01), "设备"="", "日志信息"="", "流程参数"=""} ("data in"), "时间标识"=w474, "设备"="系统", "日志信息"="平台反控变更【运行间隔】") -> (w475:T3)
                n293 = call "日志存储 (子VI).vi"("data in"=w475) -> ()  [unwired: 11 in]
              }
            }
          }
          frame #1 {
            n294 = Wait (ms)(milliseconds to wait=u32 500 ("等待时间（毫秒）")) -> ()  [unwired: 1 out]
          }
          frame #2 {
            "register values" <- w496
          }
        }
        n295 = Array Subset(array=w69, length=6 ("长度")) -> (→"系统启动命令":u16[])  [unwired: 1 in]
        n296 = Array Subset(array=w69, index=30 ("索引"), length=6 ("长度")) -> (→"单仪器启动命令":u16[])
        n297 = Array Subset(array=w69, index=14 ("索引"), length=1 ("长度")) -> (→"运行周期":u16[])
      }
      frame "写入" {
      }
    }
    n298 = Wait (ms)(milliseconds to wait=u32 1000 ("等待时间（毫秒）")) -> ()  [unwired: 1 out]
  }
  n299 = call-dynamic "Shutdown.vi"("error in"=w13, "Modbus slave in"=w14) -> ()  [unwired: 9 in, 1 out]
